vi "sub_strain-calsum.vi"(11 "data":waveform(dbl)[](array[waveform])) -> (2 "caFwf":waveform(dbl)[](array[waveform]), 3 "rawFwf":waveform(dbl)[](array[waveform]))   [LabVIEW 2013]
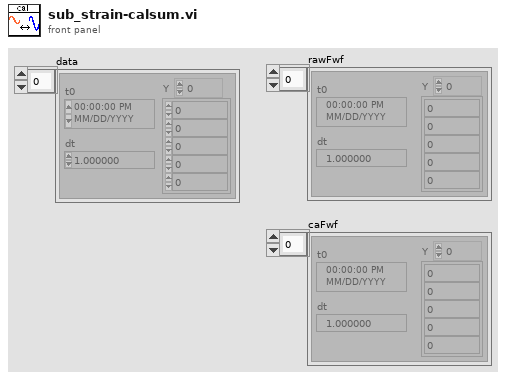
[diagram p1: front panel]
types:
  T1 = typedef "config_ctl.ctl" = cluster{"Trigger minlevel":dbl, "Lower Cut-Off":dbl, "Vacuum Trigger level":dbl, "state settings":cluster{"method":enum32{"histogram", "peak", "auto select"}, "histogram size":i32, "histogram method":enum16{"mode"}, "reserved":dbl}, "SPA-300 Setting":cluster{"Bonding force (g)":dbl, "Bonding time (ms)":dbl, "Pickup force (g)":dbl, "Pickup time (ms)":dbl, "Speed":enum16{"Slow", "Fast"}}}
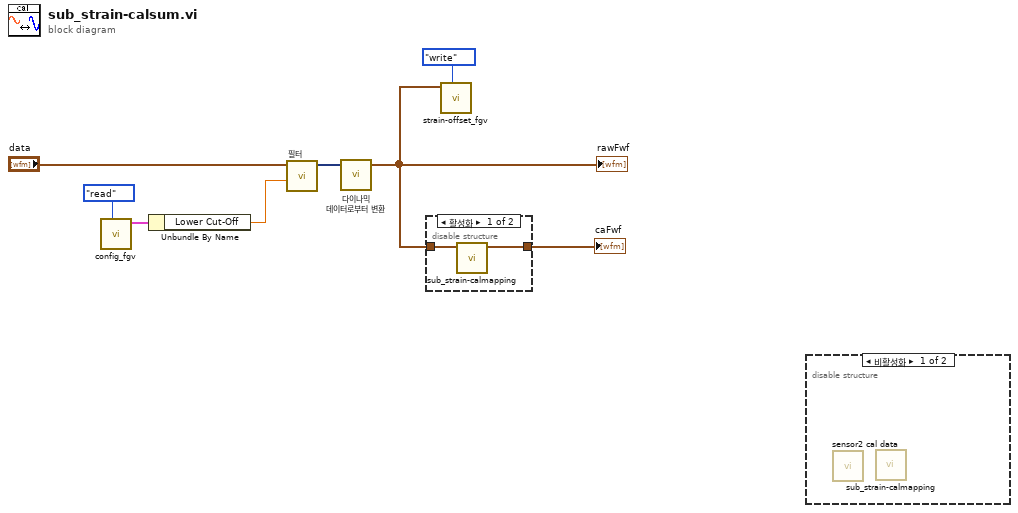
[diagram p0: block diagram]
diagram:
  n1 = call "config_fgv.vi"("cmd"=enum16{"write", "read", "ini"}."read") -> ("Config out"=w7:T1)  [unwired: 9 in, 1 out]
  n2 = Unbundle By Name(w7) -> ("Lower Cut-Off"=w4:dbl)
  n3 = call "필터"("Lower Cut-Off"=w4, "Signal"="data") -> ("Filtered Signal"=w5:dynamicdata)  [unwired: 8 in, 1 out]
  n4 = call "다이나믹 데이터로부터 변환"("Dynamic Data Type"=w5) -> ("Array of Waveform"=w1:waveform(dbl)[])  [unwired: 3 in]
  "rawFwf" <- w1
  n5 = disable-structure shown="활성화" {
    disable-tunnel: w1 -> [w10 _]
    disable-tunnel: [w9 _] -> w3
    frame Enabled {
      n6 = call "sub_strain-calmapping.vi"("input"=w10) -> ("output"=w9:waveform(dbl)[])  [unwired: 10 in]
    }
    frame Disabled {
    }
  }
  "caFwf" <- w3
  n7 = call "strain-offset_fgv.vi"("cmd"=enum16{"ini", "write", "read"}."write", "data"=w1) -> ()  [unwired: 9 in, 1 out]
  n8 = disable-structure shown="비활성화" {
    frame Disabled {
      n9 = call "sensor2 cal data.vi"() -> ()  [unwired: 11 in, 1 out]
      n10 = call "sub_strain-calmapping.vi"() -> ()  [unwired: 11 in, 1 out]
    }
    frame Enabled {
    }
  }
